vi "Viewer.vi"(9 "SetList VariableManager ref":refnum<vi>, 10 "SetList Clipboard ref":refnum<vi>) -> ()   [LabVIEW 2013]
uses:
  DeviceVIs/Device/Device.lvclass
  ColumnVIs/Column/Column.lvclass
  VariableManagerCodes/VariableManager/VariableManager.lvclass
  VariableManagerCodes/API/VariableManagerAPI.lvlib
panel:
  out "SetList Procedure Name":string
  in  "quit":bool
  out "SetList Version":string
  in  "Load Path":path
  in  "Tab Control":T1(tab)
  in  "FitCol2Text Button":bool
  in  "ManageDevicesButton":bool
  in  "Select Layout":i32(ring)=-1 items=["(On-the-fly)"=-2, "All"=-1]
  in  "Viewer Table":string[][](table)
  out "Viewer: User Functions":string
  in  "Viewer VariableManager.lvclass":refnum<class "VariableManager.lvclass">
  out "View Dev queue":refnum<queue>
  out "Col array":refnum<class "Column.lvclass">[](array[class])
  out "DevNums":i32[](array[numeric])
  in  "Devices":refnum<class "Device.lvclass">[](array[class])
  # "SetList Viewer (Read-only)"
  # "SetList references"
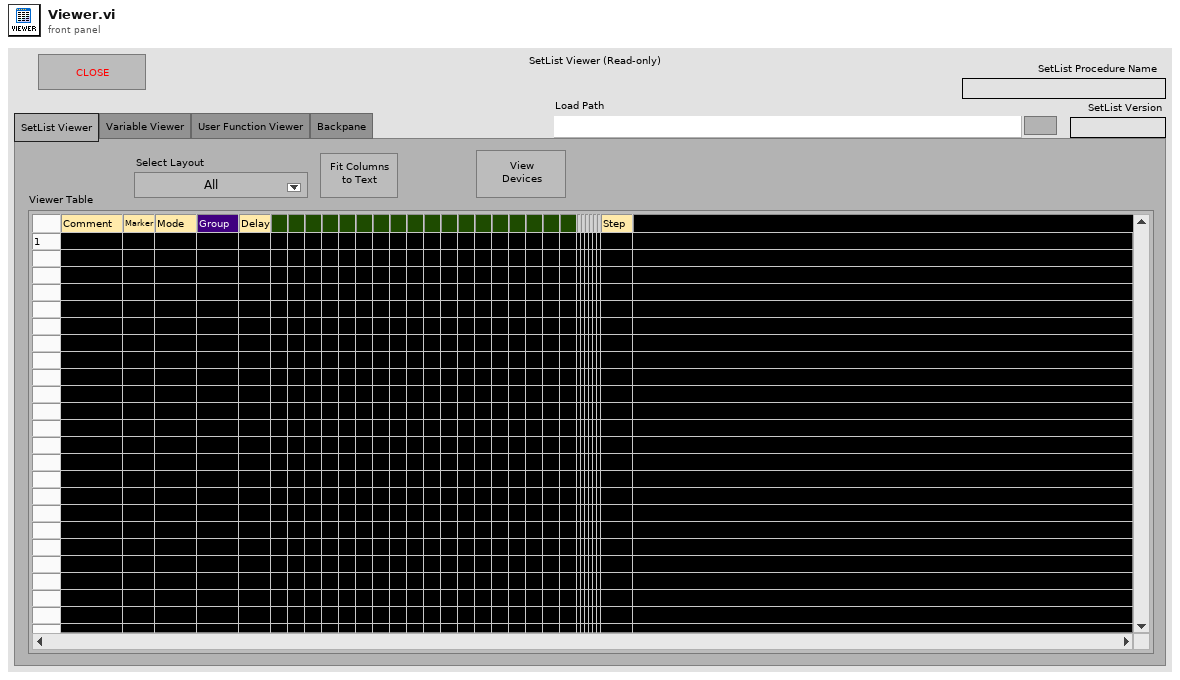
[diagram p1: front panel]
types:
  T1 = enum32{"SetList Viewer", "Variable Viewer", "User Function Viewer", "Backpane"}
  T2 = typedef "SaveCluster.ctl" = cluster{"Version":string, "Devices":refnum<class "Device.lvclass">[], "Select Layout":i32, "Layout:Strings And Values []":T3, "User defined functions":string, "VariableManager":refnum<class "VariableManager.lvclass">}
  T3 = typedef "LVStringsAndValuesArrayTypeDef_I32.ctl" = cluster{"String":string, "Value":i32}[]
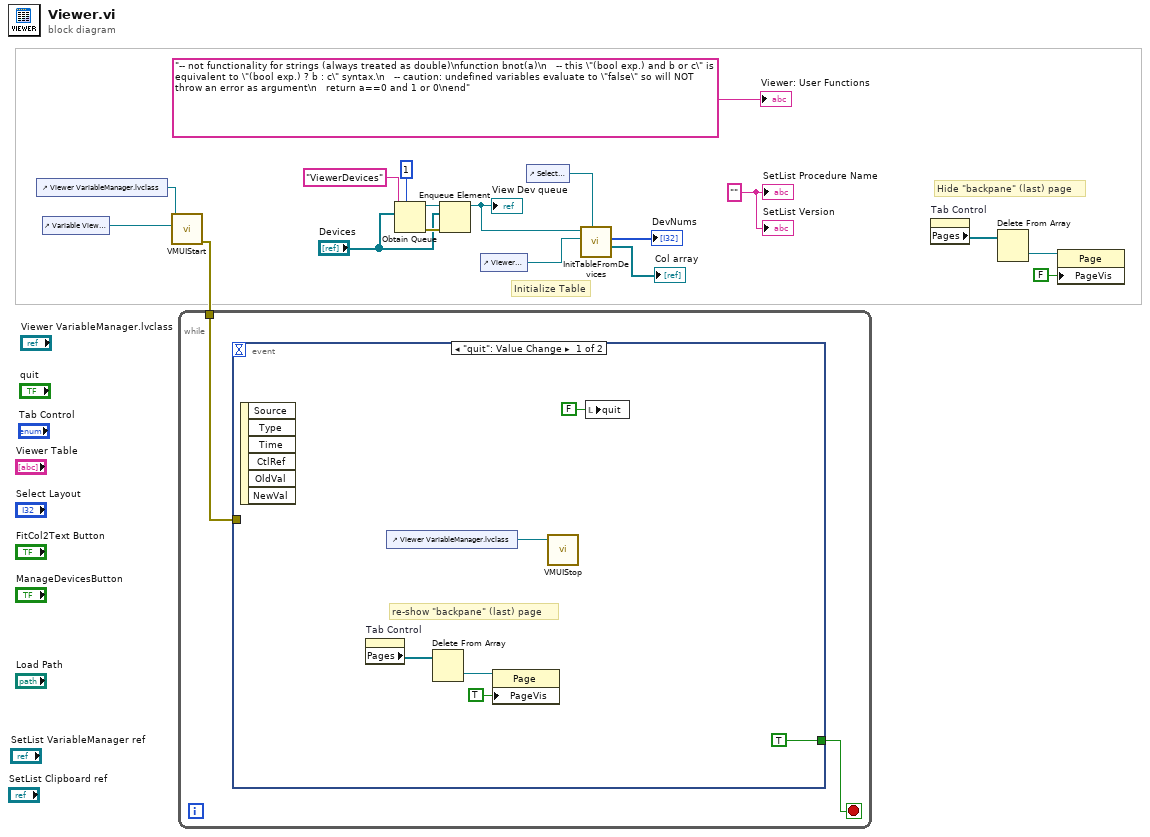
[diagram p0: block diagram]
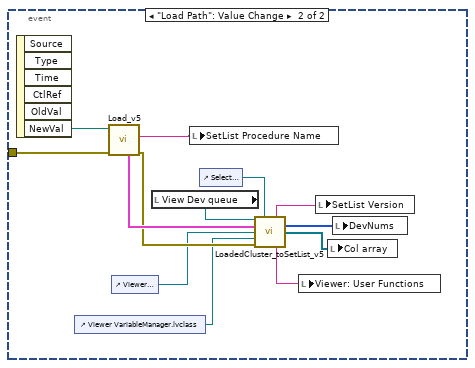
[diagram p2: hidden frame]
diagram:
  w8 = "" ("SetList Procedure Name")
  # "Hide \"backpane\" (last) page"
  # "Initialize Table"
  n1 = control-ref of="Viewer VariableManager.lvclass"() -> (w5:refnum<vi>)
  n2 = control-ref of="Variable View Pane"() -> (w6:refnum<vi>)
  n3 = call "VMUIStart.vi"("SubPanelRef"=w6, "VariableManagerRef in"=w5) -> ("error out"=w4:errorcluster)  [unwired: 8 in, 1 out]
  n4 = while {
    tunnel: w4 -> [w19]
    stop <- w20 stop-if-true
    n5 = event shown="[0] \"quit\": Value Change" {
      selector: _ -> [_ _]
      dyn-events: _ -> [_ _]
      timeout: _ -> [_ _]
      tunnel: [TRUE _] -> w20
      tunnel: w19 -> [_ w28]
      event "quit": Value Change {
        # "re-show \"backpane\" (last) page"
        n6 = event-data() -> ()  [unwired: 1 in, 6 out]
        n7 = property on="Tab Control" class="TabCtl (strict)"() -> ("Pages"=w23:refnum<vi>[])  [unwired: 2 in, 2 out]
        n8 = control-ref of="Viewer VariableManager.lvclass"() -> (w24:refnum<vi>)
        n9 = Delete From Array(array=w23) -> (deleted portion=w22:refnum<vi>)  [unwired: 2 in, 1 out]
        n10 = property class="Page"(reference=w22, "PageVis"=TRUE ("Page Visible")) -> ()  [unwired: 1 in, 2 out]
        n11 = call "VMUIStop.vi"("VariableManagerRef in"=w24) -> ()  [unwired: 9 in, 2 out]
        n12 = local write "quit"(FALSE ("quit")) -> ()
      }
      event "Load Path": Value Change {
        n13 = event-data() -> ("NewVal"=w39:path)  [unwired: 1 in, 5 out]
        n14 = control-ref of="Viewer VariableManager.lvclass"() -> (w27:refnum<vi>)
        n15 = call "Load_v5.vi"("error in"=w28, "Path (open dialog)"=w39) -> ("error out"=w37:errorcluster, "Procedure Name"=w34:string, "Save Cluster"=w38:T2)  [unwired: 5 in, 2 out]
        n16 = control-ref of="Viewer Table"() -> (w35:refnum<vi>)
        n17 = local read "View Dev queue"() -> (w30:refnum<queue>)
        n18 = local write "SetList Procedure Name"(w34) -> ()
        n19 = control-ref of="Select Layout"() -> (w36:refnum<vi>)
        n20 = call "LoadedCluster_toSetList_v5.vi"("Devices queue"=w30, "Layout Ref"=w36, "Save Cluster"=w38, "Table Ref in"=w35, "VariableManagerRef"=w27, "error in (no error)"=w37) -> ("Loaded Version"=w33:string, "DevNums"=w31:i32[], "Col array"=w32:refnum<class "Column.lvclass">[], "User defined functions"=w29:string)  [unwired: 4 in, 2 out]
        n21 = local write "Viewer: User Functions"(w29) -> ()
        n22 = local write "SetList Version"(w33) -> ()
        n23 = local write "Col array"(w32) -> ()
        n24 = local write "DevNums"(w31) -> ()
      }
    }
  }
  n25 = Obtain Queue(max queue size (-1, unlimited)=1, name (unnamed)="ViewerDevices", element data type="Devices") -> (queue out=w16:refnum<queue>, error out=w15:errorcluster)  [unwired: 2 in, 1 out]
  n26 = Enqueue Element(queue=w16, element="Devices", error in (no error)=w15) -> (queue out=w13:refnum<queue>)  [unwired: 1 in, 2 out]
  "View Dev queue" <- w13
  n27 = control-ref of="Viewer Table"() -> (w9:refnum<vi>)
  n28 = control-ref of="Select Layout"() -> (w10:refnum<vi>)
  n29 = call "InitTableFromDevices.vi"("Layout Ref"=w10, "Table Ref in"=w9, "Devices queue"=w13) -> ("Col array"=→"Col array":refnum<class "Column.lvclass">[], "DevNums"=→"DevNums":i32[])  [unwired: 5 in, 2 out]
  n30 = property on="Tab Control" class="TabCtl (strict)"() -> ("Pages"=w1:refnum<vi>[])  [unwired: 2 in, 2 out]
  n31 = Delete From Array(array=w1) -> (deleted portion=w2:refnum<vi>)  [unwired: 2 in, 1 out]
  n32 = property class="Page"(reference=w2, "PageVis"=FALSE ("Page Visible")) -> ()  [unwired: 1 in, 2 out]
  "SetList Procedure Name" <- w8
  "SetList Version" <- w8
  "Viewer: User Functions" <- "-- not functionality for strings (always treated as double)\nfunction bnot(a)\n   -- this \"(bool exp.) and b or c\" is equivalent to \"(bool exp.) ? b : c\" syntax.\n   -- caution: undefined variables evaluate to \"false\" so will NOT throw an error as argument\n   return a==0 and 1 or 0\nend" ("Viewer: User Functions")
